vi "Convert Digital Measurement to Digital PWM values.vi"(1 "Digital PWM Measurement in":T1) -> (0 "Digital PWM Values out":dbl[](array[numeric]))   [LabVIEW 2018, in "FPGA Addon Engine.lvlib"]
uses:
  FPGA Addon Engine.lvlib
  Submodules/Source/Types/PWM.Measure.Digital.Measurement.ctl
  Submodules/Source/Speciality FPGA IO.lvlib
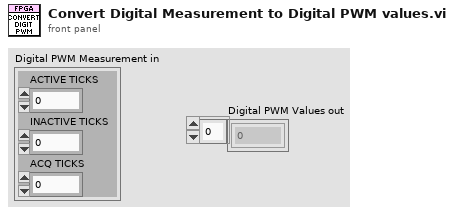
[diagram p1: front panel]
types:
  T1 = typedef "Speciality FPGA IO.lvlib/PWM.Measure.Digital.Measurement.ctl" = cluster{"ACTIVE TICKS":u32, "INACTIVE TICKS":u32, "ACQ TICKS":u32}
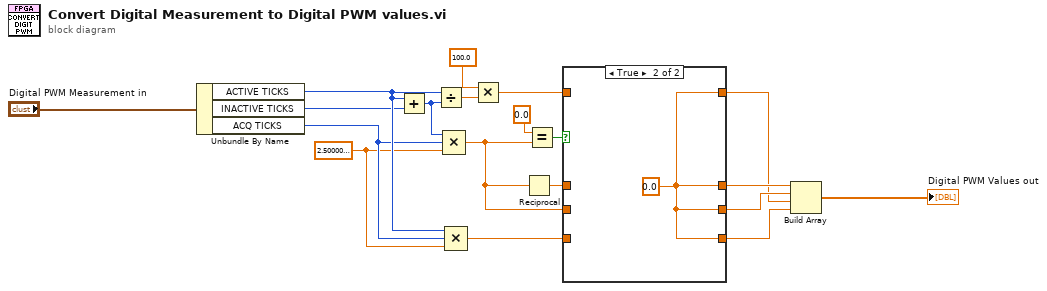
[diagram p0: block diagram]
diagram:
  w5 = 2.5000000292152436e-08 ("y")
  n1 = Unbundle By Name("Digital PWM Measurement in") -> ("ACTIVE TICKS"=w18:u32, "INACTIVE TICKS"=w15:u32, "ACQ TICKS"=w9:u32)
  n2 = Add(x=w18, y=w15) -> (x+y=w3:u32)
  n3 = Divide(x=w18, y=w3) -> (x/y=w10:dbl)
  n4 = Compound Arithmetic op=MULTIPLY(w3, w9, w5) -> (w2:dbl)
  n5 = Compound Arithmetic op=MULTIPLY(w18, w9, w5) -> (w4:dbl)
  n6 = Multiply(x=100.0, y=w10) -> (x*y=w11:dbl)
  n7 = Reciprocal(x=w2) -> (1/x=w1:dbl)
  n8 = Equal?(x=0.0, y=w2) -> (x = y?=w6:bool)
  n9 = case shown="True" w6 {
    tunnel: [w20 w24] -> w16
    tunnel: [w21 w24] -> w14
    tunnel: [w23 w24] -> w17
    tunnel: w2 -> [w23 _]
    tunnel: [w22 w24] -> w12
    tunnel: w4 -> [w22 _]
    tunnel: w11 -> [w21 _]
    tunnel: w1 -> [w20 _]
    frame False {
    }
    frame True {
      w24 = 0.0 ("x")
    }
  }
  n10 = Build Array(w16, w17, w14, w12) -> (→"Digital PWM Values out":dbl[])
